vi "Select Device.vi"(8 "Error In":errorcluster, 11 "Test Framework.lvclass":refnum<class "Test Framework.lvclass">) -> (0 "Error Out":errorcluster, 3 "Test Framework out":refnum<class "Test Framework.lvclass">)   [LabVIEW 2020, in "Test Framework.lvclass"]
uses:
  Test Framework.lvclass
  Test Framework.lvclass/Test Framework.ctl
  Devices/PIC-device/PIC-Device.lvclass
  Devices/PIC-device/PIC-Device.lvclass/PIC-Device.ctl
  Devices/Device.lvclass
panel:
  in  "Cancel Button":bool
  in  "Settings Button":bool
  out "Current Device":string
  in  "Device":u16(ring) items=["WS1021", "CK", "Maxscend SP4T", "Qorvo QM13xxx", "WS5100", "Toggle 8 (niDig)", "Thru", "WS1040", "WS1041", "WS1042", "WS1050 1.1", "WS1051 1.1"]
  in  "OK Button":bool
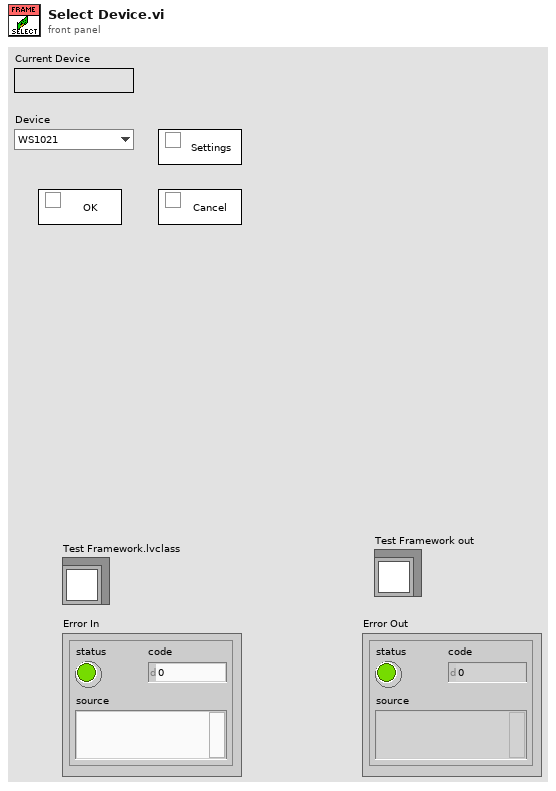
[diagram p1: front panel]
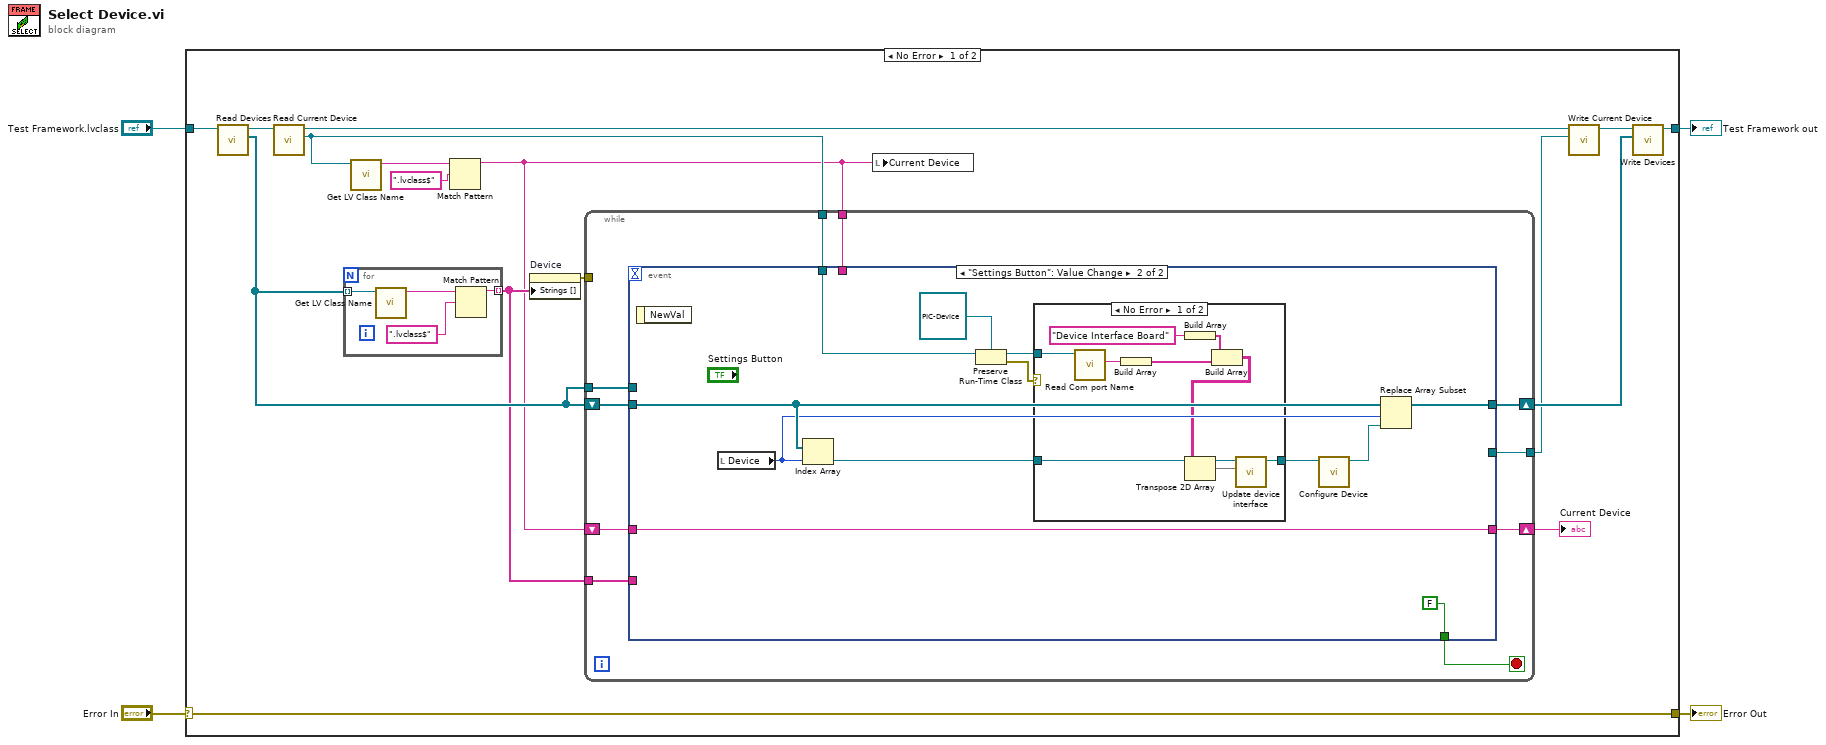
[diagram p0: block diagram]
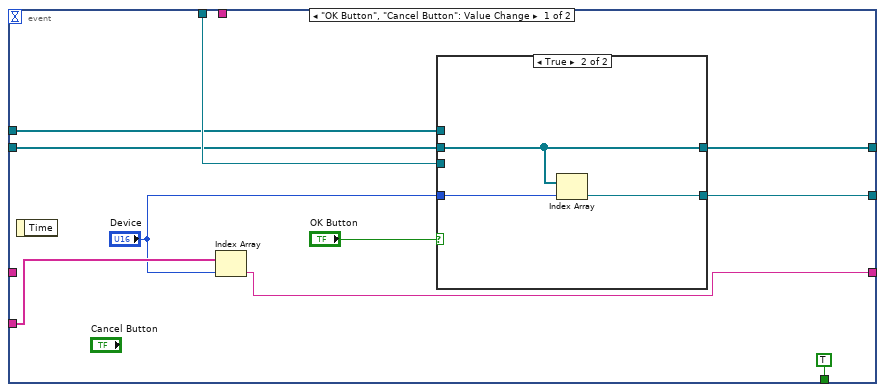
[diagram p2: hidden frame]
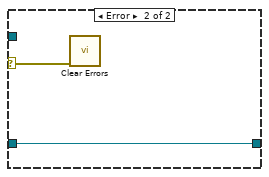
[diagram p4: hidden frame]
diagram:
  n1 = case shown="No Error" "Error In" {
    selector: "Error In" -> [w14 w74]
    tunnel: [w14 w74] -> w3
    tunnel: "Test Framework.lvclass" -> [w20 w73]
    tunnel: [w15 w73] -> w1
    frame No Error {
      n2 = call "Read Devices.vi"("Test Framework in"=w20) -> ("Devices"=w8:refnum<class "Device.lvclass">[], "Test Framework out"=w18:refnum<class "Test Framework.lvclass">)  [unwired: 9 in]
      n3 = call-dynamic "Read Current Device.vi"("Test Framework in"=w18) -> ("Current Device.lvclass"=w10:refnum<class "Device.lvclass">, "Test Framework out"=w17:refnum<class "Test Framework.lvclass">)  [unwired: 9 in]
      n4 = for {
        tunnel: w8 -> [w72] mode=indexing
        tunnel: [w69] -> w7 mode=indexing
        n5 = call <vilib>:"Get LV Class Name.vi"("object"=w72) -> ("class name"=w71:string)  [unwired: 9 in, 1 out]
        n6 = Match Pattern(string=w71, regular expression=".lvclass$") -> (before substring=w69:string)  [unwired: 1 in, 3 out]
      }
      n7 = call <vilib>:"Get LV Class Name.vi"("object"=w10) -> ("class name"=w13:string)  [unwired: 9 in, 1 out]
      n8 = Match Pattern(string=w13, regular expression=".lvclass$") -> (before substring=w6:string)  [unwired: 1 in, 3 out]
      n9 = property on="Device" class="Ring (strict)"("Strings []"=w7) -> (error out=w19:errorcluster)  [unwired: 2 in, 1 out]
      n10 = while {
        tunnel: w19 -> [_]
        tunnel: w7 -> [w29]
        shift-right: [w23] -> w9
        shift-left: w6 -> [w28]
        tunnel: w6 -> [w27]
        tunnel: w10 -> [w25]
        shift-right: [w24] -> w11
        shift-left: w8 -> [w26]
        tunnel: w8 -> [w22]
        tunnel: [w21] -> w5
        stop <- w30 stop-if-true
        n11 = event shown="[1] \"Settings Button\": Value Change" {
          selector: _ -> [_ _]
          dyn-events: _ -> [_ _]
          timeout: _ -> [_ _]
          tunnel: [TRUE FALSE] -> w30
          tunnel: w27 -> [_ _]
          tunnel: [w37 _] -> w21
          tunnel: w29 -> [w35 _]
          tunnel: [w34 w56] -> w23
          tunnel: w28 -> [_ w56]
          tunnel: w26 -> [w33 w55]
          tunnel: w25 -> [w39 w52]
          tunnel: [w38 w54] -> w24
          tunnel: w22 -> [w32 _]
          event "OK Button", "Cancel Button": Value Change {
            n12 = event-data() -> ()  [unwired: 1 in, 1 out]
            n13 = Index Array(array=w35, index="Device") -> (element=w34:string)
            n14 = case shown="True" "OK Button" {
              tunnel: w33 -> [_ w45]
              tunnel: [w41 w45] -> w38
              tunnel: w39 -> [w42 _]
              tunnel: [w42 w43] -> w37
              tunnel: w32 -> [w41 _]
              tunnel: "Device" -> [_ w44]
              frame False {
              }
              frame True {
                n15 = Index Array(array=w45, index=w44) -> (element=w43:refnum<class "Device.lvclass">)
              }
            }
          }
          event "Settings Button": Value Change {
            n16 = event-data() -> ()  [unwired: 1 in, 1 out]
            n17 = local read "Device"() -> (w53:u16)
            n18 = Index Array(array=w55, index=w53) -> (element=w46:refnum<class "Device.lvclass">)
            n19 = Preserve Run-Time Class(object in=w52, 2:refnum<class "PIC-Device.lvclass"> refnum ("PIC-Device.lvclass")) -> (object out=w50:refnum<class "PIC-Device.lvclass">, error out=w49:errorcluster)  [unwired: 1 in]
            n20 = case shown="No Error" w49 {
              selector: w49 -> [_ w68]
              tunnel: w46 -> [w66 w67]
              tunnel: [w65 w67] -> w48
              tunnel: w50 -> [w64 _]
              frame No Error {
                n21 = call "Read Com port Name.vi"("Device in"=w64) -> ("Com port Name"=w61:string)  [unwired: 9 in, 1 out]
                n22 = Build Array(w61) -> (w60:string[])
                n23 = Build Array("Device Interface Board") -> (w63:string[])
                n24 = Build Array(w63, w60) -> (w59:string[][])
                n25 = Transpose 2D Array(2D array=w59) -> (transposed array=w58:string[][])
                n26 = call-dynamic "Update device interface.vi"("Found Instruments"=w58, "Device in"=w66) -> ("Device out"=w65:refnum<class "Device.lvclass">)  [unwired: 8 in, 1 out]
              }
              frame Error {
                n27 = call <vilib>:"Clear Errors.vi"("error in (no error)"=w68) -> ()  [unwired: 5 in, 2 out]
              }
            }
            n28 = call-dynamic "Configure Device.vi"("Device in"=w48) -> ("Device out"=w47:refnum<class "Device.lvclass">)  [unwired: 9 in, 1 out]
            n29 = Replace Array Subset(array=w55, new element=w47, index=w53) -> (w54:refnum<class "Device.lvclass">[])
          }
        }
      }
      "Current Device" <- w9
      n30 = local write "Current Device"(w6) -> ()
      n31 = call-dynamic "Write Current Device.vi"("Current Device.lvclass"=w5, "Test Framework in"=w17) -> ("Test Framework out"=w16:refnum<class "Test Framework.lvclass">)  [unwired: 9 in]
      n32 = call "Write Devices.vi"("Devices"=w11, "Test Framework in"=w16) -> ("Test Framework out"=w15:refnum<class "Test Framework.lvclass">)  [unwired: 9 in]
    }
    frame Error {
    }
  }
  "Error Out" <- w3
  "Test Framework out" <- w1
